vi "Connect.vi"(8 "error in":errorcluster, 11 "MPLab in":refnum<class "MPLab.lvclass">) -> (0 "error out":errorcluster, 3 "MPLab out":refnum<class "MPLab.lvclass">)   [LabVIEW 2018, in "MPLab.lvlib" / "MPLab.lvclass"]
uses:
  MPLab.lvclass
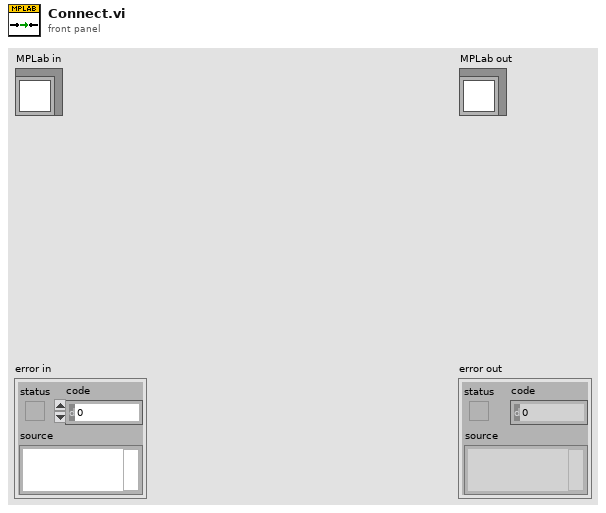
[diagram p1: front panel]
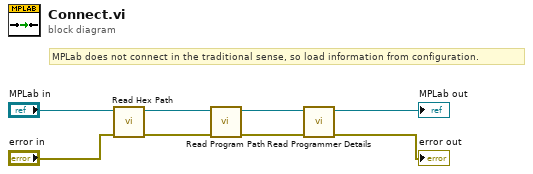
[diagram p0: block diagram]
diagram:
  # "MPLab does not connect in the traditional sense, so load information from configuration."
  n1 = call "Read Hex Path.vi"("error in"="error in", "MPLab in"="MPLab in") -> ("error out"=w7:errorcluster, "MPLab out"=w8:refnum<class "MPLab.lvclass">)  [unwired: 8 in]
  n2 = call "Read Program Path.vi"("error in"=w7, "MPLab in"=w8) -> ("error out"=w2:errorcluster, "MPLab out"=w4:refnum<class "MPLab.lvclass">)  [unwired: 8 in]
  n3 = call "Read Programmer Details.vi"("error in"=w2, "MPLab in"=w4) -> ("error out"=→"error out":errorcluster, "MPLab out"=→"MPLab out":refnum<class "MPLab.lvclass">)  [unwired: 8 in]
